vi "Volts to I16.vi"(7 "Voltage (V)":dbl=20.0 format="%#_13g", 11 "Volatge (I16)":i16=20) -> (8 "I16":i16, 15 "Voltage (V)":dbl)   [LabVIEW 2014]
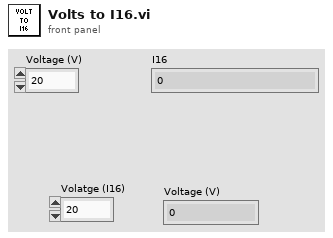
[diagram p1: front panel]
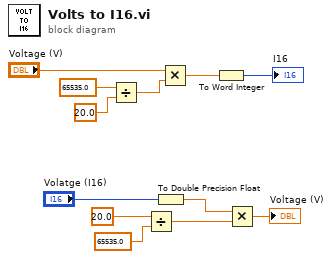
[diagram p0: block diagram]
diagram:
  n1 = Divide(x=65535.0, y=20.0 ("x")) -> (x/y=w10:dbl)
  n2 = Divide(x=20.0, y=65535.0 ("x")) -> (x/y=w4:dbl)
  n3 = To Double Precision Float(number="Volatge (I16)") -> (double precision float=w1:dbl)
  n4 = Multiply(x="Voltage (V)", y=w10) -> (x*y=w8:dbl)
  n5 = To Word Integer(number=w8) -> (16bit integer=→"I16":i16)
  n6 = Multiply(x=w1, y=w4) -> (x*y=→"Voltage (V)":dbl)
